vi "Init.vi"(8 "error in (no error)":errorcluster, 11 "Result Table in":refnum<class "Result Table.lvclass">) -> (0 "error out":errorcluster, 2 "Result Texts":string[](array[string]), 3 "Result Table out":refnum<class "Result Table.lvclass">)   [LabVIEW 2020, in "Result Table.lvclass"]
uses:
  Result Table.lvclass
  Private/TypeDefs/Results.ctl
  Result Table.lvclass/Result Table.ctl
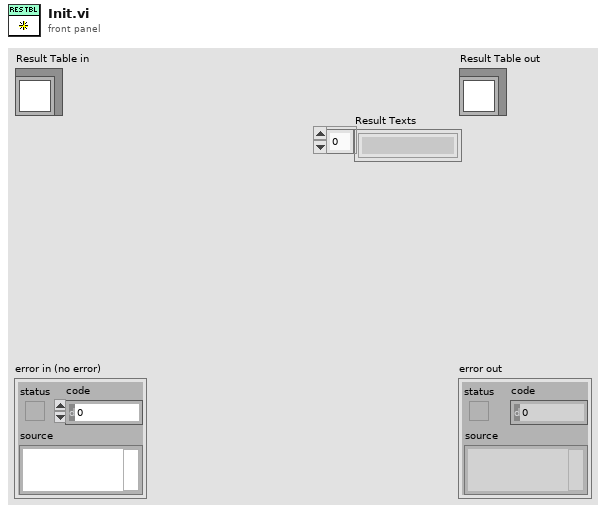
[diagram p1: front panel]
types:
  T1 = typedef "Result Table.lvclass/Results.ctl" = cluster{"Method Count":u32, "Executed Methods":u32, "Passed Methods":u32, "Failed Methods":u32, "Method Errors":u32, "Skipped Method":u32}
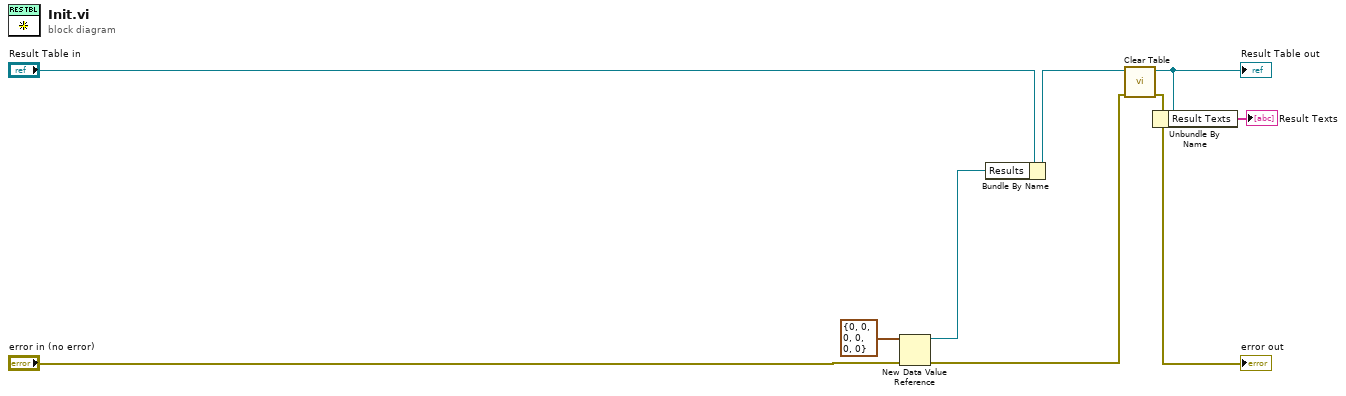
[diagram p0: block diagram]
diagram:
  n1 = New Data Value Reference(data value=T1 {"Method Count"=0, "Executed Methods"=0, "Passed Methods"=0, "Failed Methods"=0, "Method Errors"=0, "Skipped Method"=0} ("Results"), error in="error in (no error)") -> (data value reference=w7:refnum<data-value>, error out=w5:errorcluster)
  n2 = Bundle By Name(cluster="Result Table in", "Results"=w7) -> (w6:refnum<class "Result Table.lvclass">)
  n3 = call "Clear Table.vi"("error in (no error)"=w5, "Result Table.lvclass"=w6) -> ("error out"=→"error out":errorcluster, "Result Table"=w2:refnum<class "Result Table.lvclass">)  [unwired: 8 in]
  "Result Table out" <- w2
  n4 = Unbundle By Name(w2) -> ("Result Texts"=→"Result Texts":string[])
